vi "StopSync.vi"(8 "error in (no error)":errorcluster, 11 "PXI_MultiTrig in":refnum<class "PXI_MultiTrig.lvclass">) -> (0 "error out":errorcluster, 3 "PXI_MultiTrig out":refnum<class "PXI_MultiTrig.lvclass">)   [LabVIEW 2018, in "SyncPlugins.lvlib" / "PXI_MultiTrig.lvclass"]
uses:
  PXI_MultiTrig.lvclass
  Y:/Projects/PMUCal/Modules/Sync/SyncPlugins/SyncPluginBase/SyncPluginBase.lvclass
  SyncPluginBase/SyncPluginBase.lvclass/SyncPluginBase.ctl
  SyncPluginBase/Accessors/Read Initiated.vi
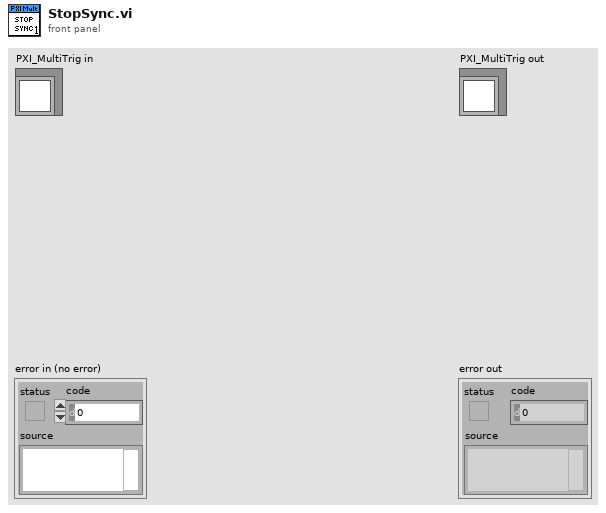
[diagram p1: front panel]
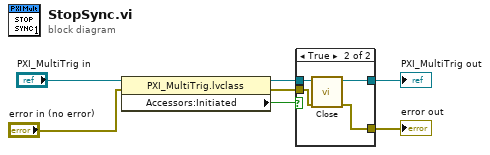
[diagram p0: block diagram]
diagram:
  n1 = property class="PXI_MultiTrig.lvclass"(reference="PXI_MultiTrig in", error in="error in (no error)") -> (reference out=w5:refnum<class "PXI_MultiTrig.lvclass">, error out=w3:errorcluster, "Accessors:Initiated"=w2:bool)
  n2 = case shown="True" w2 {
    tunnel: [w9 w13] -> w7
    tunnel: [w8 w12] -> w1
    tunnel: w5 -> [w9 w11]
    tunnel: w3 -> [w8 w10]
    frame False {
    }
    frame True {
      n3 = call-dynamic "Close.vi"("error in (no error)"=w10, "PXI_MultiTrig in"=w11) -> ("error out"=w12:errorcluster, "PXI_MultiTrig out"=w13:refnum<class "PXI_MultiTrig.lvclass">)  [unwired: 8 in]
    }
  }
  "error out" <- w1
  "PXI_MultiTrig out" <- w7
